vi "Database Query Timing.vi"(8 "error in (no error)":errorcluster, 9 "Requesting Module":T1, 10 "Requested Step":T2, 11 "Status":T3) -> (0 "error out":errorcluster, 3 "Status":T3)   [LabVIEW 2016]
doc: "Allow access to timing information for each step"
uses:
  Controls/Database Status.ctl
  Architecture/Message Queue/Message Cluster.ctl
  Car Wash Controller/Controls/Steps.ctl
  Car Wash Controller/Controls/Stations.ctl
  Architecture/Modules.ctl
  Architecture/Message Queue/Message Queue.lvlib
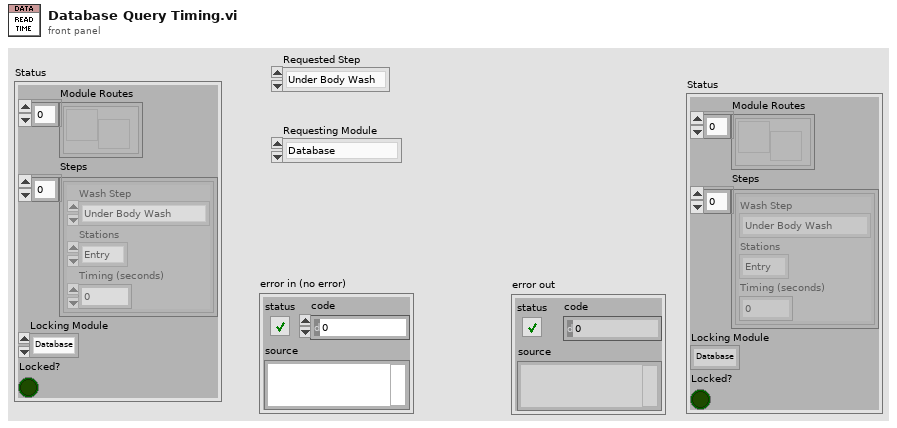
[diagram p1: front panel]
types:
  T1 = typedef "Modules.ctl" = enum16{"Database", "Car Wash Controller", "Console"}
  T2 = typedef "Steps.ctl" = enum16{"Under Body Wash", "Bug Remover", "Pre-Soak", "High Pressure Wash", "Low Pressure Wax", "Spot Free Rinse", "Tire Shine Foam", "Air Dry"}
  T3 = typedef "Database Status.ctl" = cluster{"Module Routes":refnum<user-event>[], "Steps":cluster{"Wash Step":T2, "Stations":T4, "Timing (seconds)":u32}[], "Locking Module":T1, "Locked?":bool}
  T4 = typedef "Stations.ctl" = enum16{"Entry", "Station 1", "Station 2", "Station 3", "Exit"}
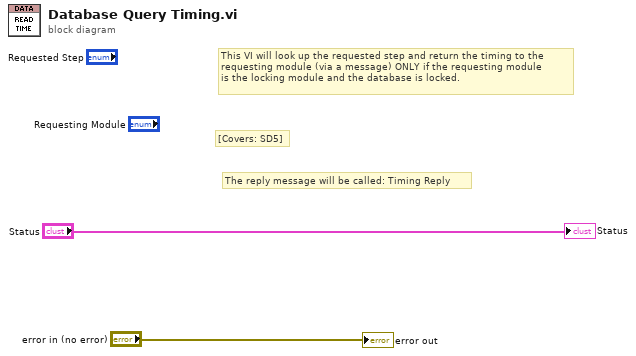
[diagram p0: block diagram]
diagram:
  # "The reply message will be called: Timing Reply"
  # "[Covers: SD5]"
  # "This VI will look up the requested step and return the timing to the\nrequesting module (via a message) ONLY if the requesting module\nis the locking module and the database is locked."
  "error out" <- "error in (no error)"
  "Status" <- "Status"
